vi "configure.vi"(8 "error in (no error)":errorcluster, 11 "GenericPlugin in":refnum<class "ClockMT120808DAQmxSimple.lvclass">) -> (0 "error out":errorcluster, 3 "GenericPlugin out":refnum<class "ClockMT120808DAQmxSimple.lvclass">)   [LabVIEW 2010, in "ClockMT120808DAQmxSimple.lvclass"]
doc: "The dynamic dispatch version of this VI loads and displays the configuration file associated with the plug-in object. The user modify and save the configuration data."
uses:
  ClockMT120808DAQmxSimple.lvclass
  ClockMT120808DAQmxSimple.lvclass/ClockMT120808DAQmxSimple.ctl
panel:
  in  "counter":tag
  in  "cancelButton":bool
  in  "saveButton":bool
  # "Configure ClockDL100201DAQmx"
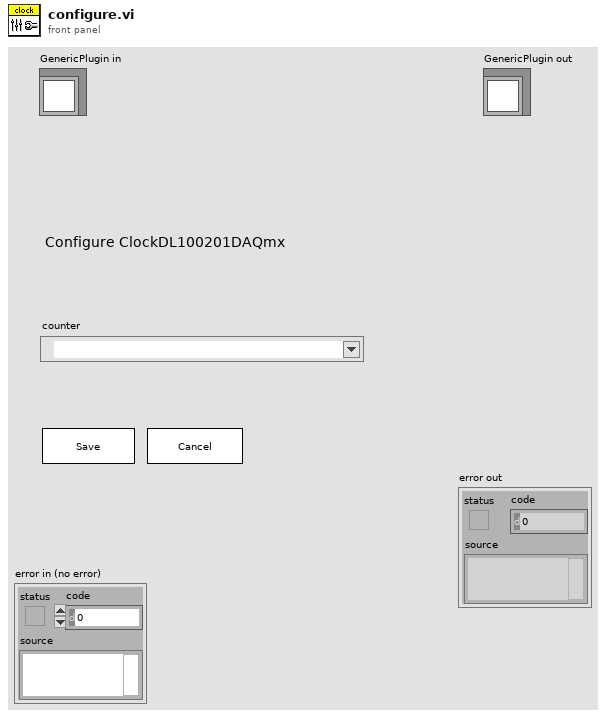
[diagram p1: front panel]
types:
  T1 = typedef "ClockMT120808DAQmxSimple.lvclass/config_data_cluster.ctl" = cluster{"counter":string}
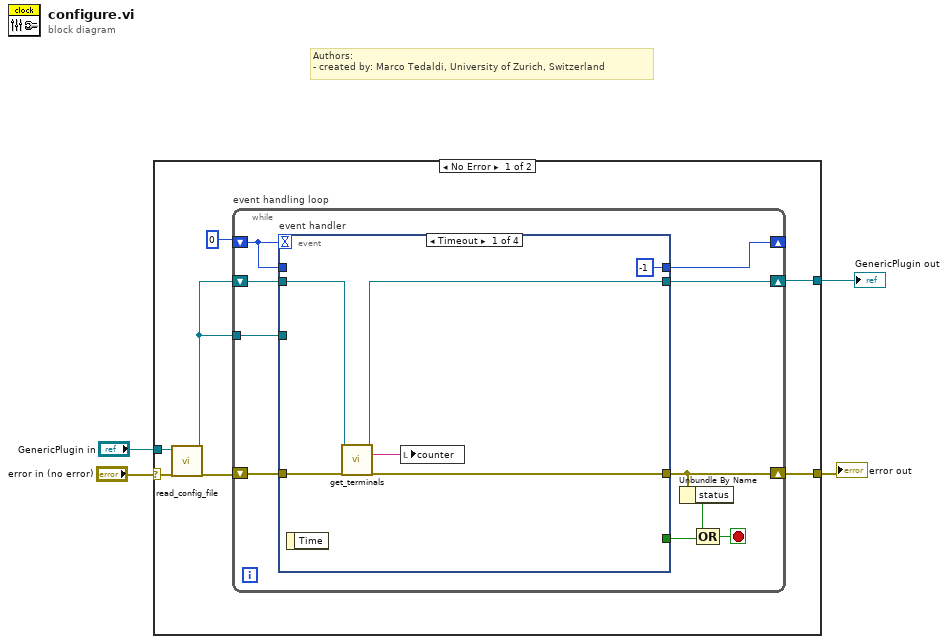
[diagram p0: block diagram]
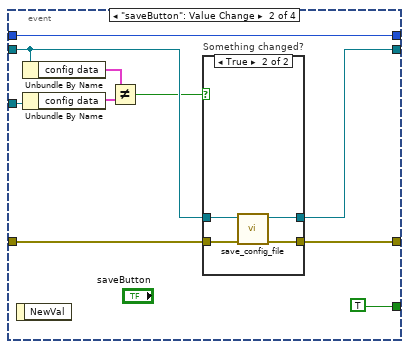
[diagram p2: hidden frame]
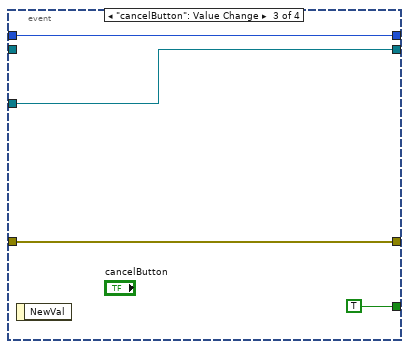
[diagram p4: hidden frame]
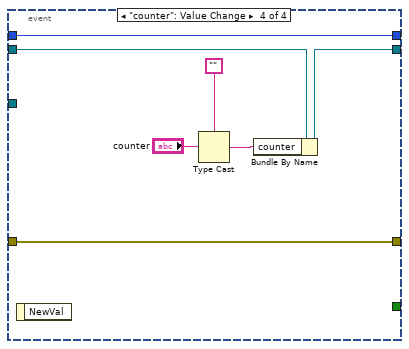
[diagram p5: hidden frame]
diagram:
  # "Authors: \n- created by: Marco Tedaldi, University of Zurich, Switzerland"
  n1 = case shown="No Error" "error in (no error)" {
    selector: "error in (no error)" -> [w8 w56]
    tunnel: [w10 w56] -> w3
    tunnel: [w9 w55] -> w2
    tunnel: "GenericPlugin in" -> [w6 w55]
    frame No Error {
      n2 = call-dynamic "read_config_file.vi"("error in (no error)"=w8, "GenericPlugin in"=w6) -> ("error out"=w7:errorcluster, "GenericPlugin out"=w5:refnum<class "ClockMT120808DAQmxSimple.lvclass">)  [unwired: 8 in]
      n3 = while "event handling loop" {
        shift-right: [w20] -> _
        shift-left: 0 -> [w21]
        shift-right: [w15] -> w10
        shift-left: w7 -> [w19]
        shift-right: [w17] -> w9
        shift-left: w5 -> [w18]
        tunnel: w5 -> [w16]
        stop <- w12 stop-if-true
        n4 = event "event handler" shown="[0] Timeout" {
          selector: _ -> [_ _ _ _]
          dyn-events: _ -> [_ _ _ _]
          timeout: w21 -> [_ _ _ _]
          tunnel: w21 -> [_ w37 w47 w54]
          tunnel: [-1 w37 w47 w54] -> w20
          tunnel: w19 -> [w26 w35 w46 w53]
          tunnel: [w25 w34 w46 w53] -> w15
          tunnel: w18 -> [w24 w32 _ w52]
          tunnel: [w23 w33 w44 w51] -> w17
          tunnel: [_ TRUE TRUE _] -> w14
          tunnel: w16 -> [_ w31 w44 _]
          event Timeout {
            n5 = event-data() -> ()  [unwired: 1 in, 1 out]
            n6 = call "get_terminals.vi"("ClockDL100201DAQmx in"=w24, "error in (no error)"=w26) -> ("ClockDL100201DAQmx out"=w23:refnum<class "ClockMT120808DAQmxSimple.lvclass">, "counter"=w22:tag, "error out"=w25:errorcluster)  [unwired: 11 in]
            n7 = local write "counter"(w22) -> ()
          }
          event "saveButton": Value Change {
            n8 = event-data() -> ()  [unwired: 1 in, 1 out]
            n9 = Unbundle By Name(w32) -> ("config data"=w28:T1)
            n10 = Unbundle By Name(w31) -> ("config data"=w30:T1)
            n11 = Not Equal?(x=w28, y=w30) -> (x != y?=w29:bool)
            n12 = case "Something changed?" shown="True" w29 {
              tunnel: w35 -> [w38 w43]
              tunnel: [w38 w42] -> w34
              tunnel: w32 -> [w39 w41]
              tunnel: [w39 w40] -> w33
              frame False {
              }
              frame True {
                n13 = call-dynamic "save_config_file.vi"("error in (no error)"=w43, "GenericPlugin in"=w41) -> ("error out"=w42:errorcluster, "GenericPlugin out"=w40:refnum<class "ClockMT120808DAQmxSimple.lvclass">)  [unwired: 8 in]
              }
            }
          }
          event "cancelButton": Value Change {
            n14 = event-data() -> ()  [unwired: 1 in, 1 out]
          }
          event "counter": Value Change {
            n15 = event-data() -> ()  [unwired: 1 in, 1 out]
            n16 = Type Cast(type="", x="counter") -> (*(type *) &x=w48:string)
            n17 = Bundle By Name(cluster=w52, "counter"=w48) -> (w51:refnum<class "ClockMT120808DAQmxSimple.lvclass">)
          }
        }
        n18 = Unbundle By Name(w15) -> ("status"=w13:bool)
        n19 = Compound Arithmetic op=OR(w13, w14) -> (w12:bool)
      }
    }
    frame Error {
    }
  }
  "error out" <- w3
  "GenericPlugin out" <- w2
